vi "CircleCenter.vi"() -> ()   [LabVIEW 2016]
uses:
  <vilib>/userdefined/High Color/IMAQdx.ctl
  <vilib>/vision/driver/NI_Vision_Acquisition_Software.lvlib
panel:
  out "?":string
  out "Image 2":T1(plugin-control)
  out "Image":T1(plugin-control)
  out "Circle Descriptor":T2(array[cluster])
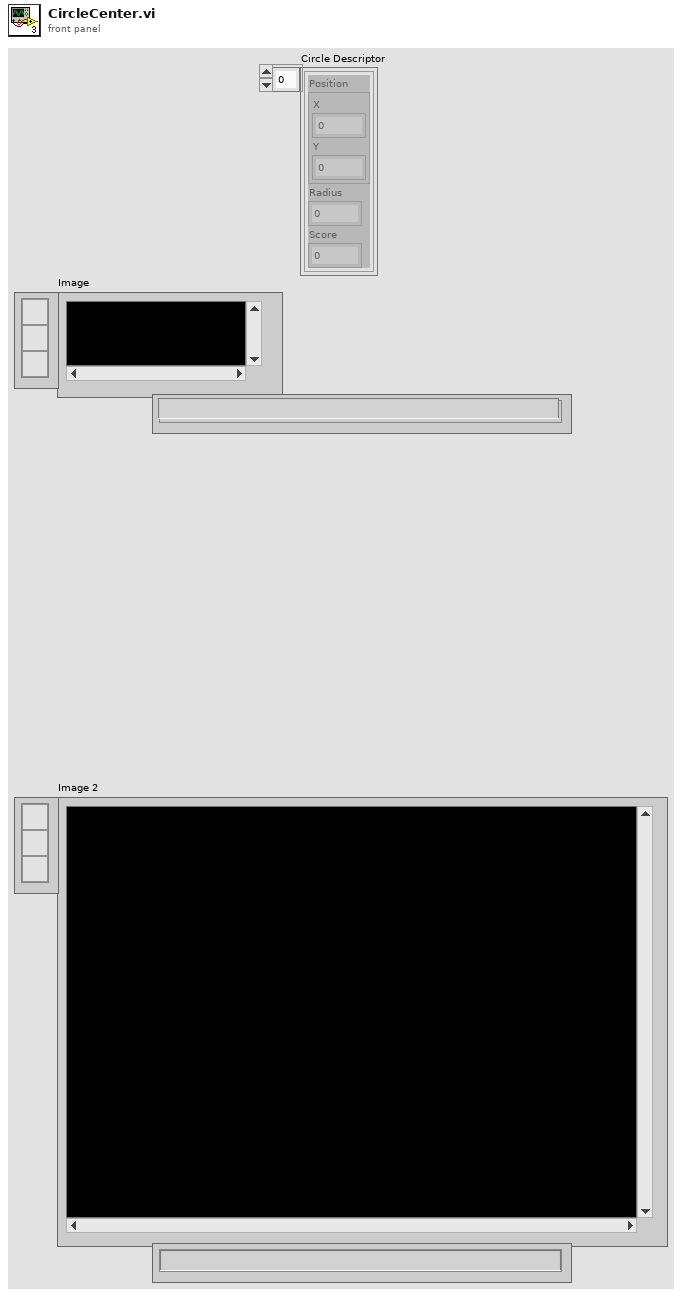
[diagram p1: front panel]
types:
  T1 = typedef "IMAQ Image.ctl" = refnum<image>
  T2 = cluster{"Position":cluster{"X":sgl, "Y":sgl}, "Radius":dbl, "Score":dbl}[]
  T3 = typedef "IMAQdx.ctl" = refnum<k21>
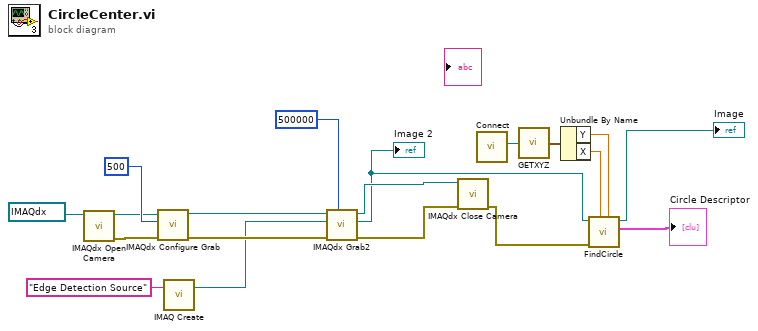
[diagram p0: block diagram]
diagram:
  n1 = call <vilib>:"IMAQdx Open Camera.vi"("Session In"=T3 "cam0") -> ("error out"=w18:errorcluster, "Session Out"=w17:T3)  [unwired: 9 in]
  n2 = call <vilib>:"IMAQdx Configure Grab.vi"("error in"=w18, "Number of Buffers"=u32 500, "Session In"=w17) -> ("error out"=w14:errorcluster, "Session Out"=w15:T3)  [unwired: 7 in]
  n3 = call "IMAQ Create"("Image Name"="Edge Detection Source") -> ("New Image"=w12:T1)  [unwired: 4 in, 1 out]
  n4 = call <vilib>:"IMAQdx Grab2.vi"("Timeout (ms)"=500000, "error in"=w14, "Image In"=w12, "Session In"=w15) -> ("error out"=w4:errorcluster, "Image Out"=w2:T1, "Session Out"=w5:T3)  [unwired: 4 in, 1 out]
  "Image 2" <- w2
  n5 = call <vilib>:"IMAQdx Close Camera.vi"("error in"=w4, "Session In"=w5) -> ("error out"=w1:errorcluster)  [unwired: 9 in]
  n6 = call "Connect.vi"() -> ("controller"=w6:refnum<k24>)  [unwired: 10 in, 1 out]
  n7 = call "GETXYZ.vi"(".NET Refnum in"=w6) -> ("XYZ"=w11:cluster{"X":dbl, "Y":dbl, "Z":dbl})
  n8 = Unbundle By Name(w11) -> ("Y"=w10:dbl, "X"=w9:dbl)
  n9 = call "FindCircle.vi"("Y"=w10, "X"=w9, "error in (no error)"=w1, "Image 2"=w2) -> ("Circle Descriptor"=→"Circle Descriptor":T2, "Image Out"=→"Image":T1)  [unwired: 5 in, 1 out]
